vi "LanchSpeedAndAngleCalculator.vi"(2 "g":dbl=9.82, 3 "b":dbl=60.0, 4 "h":dbl, 5 "d":dbl) -> (0 "V":dbl, 1 "a":dbl)   [LabVIEW 2011]
uses:
  <vilib>/express/express arith-compare/Formula/XNode/ExpressFormulaBlockNode.xnode
panel:
  # "a - degrees\nb - degrees\nh - meters\nd - meters\ng - m/s^2\nV - m/s"
  # "b"
  # "V"
  # "h"
  # "a"
  # "d"
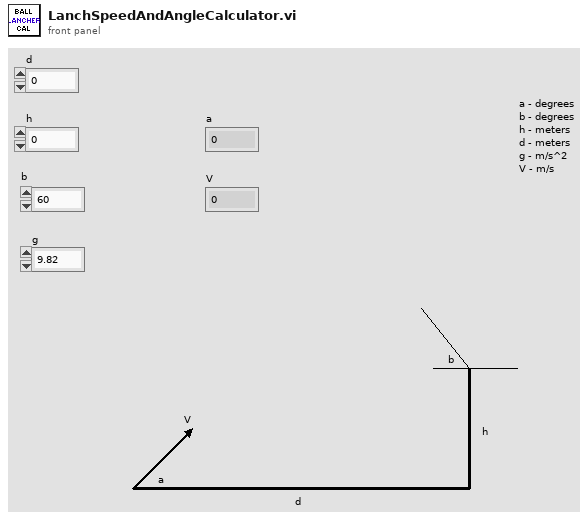
[diagram p1: front panel]
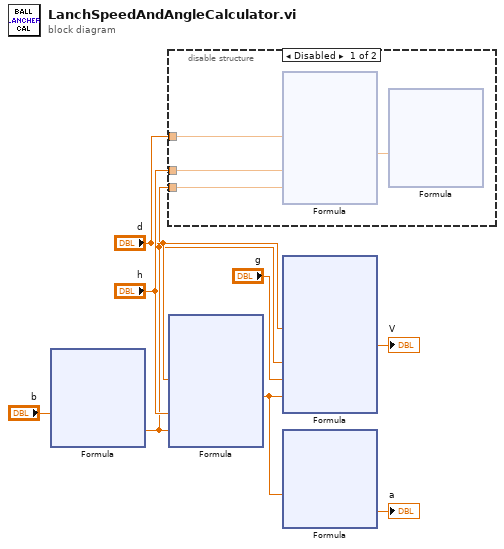
[diagram p0: block diagram]
diagram:
  n1 = xnode "Formula"("b"="b") -> ("Result"=w1:dbl)  [unwired: 1 in, 1 out]
  n2 = disable-structure shown="Disabled" {
    disable-tunnel: "d" -> [w12 _]
    disable-tunnel: "h" -> [w11 _]
    disable-tunnel: w1 -> [w10 _]
    frame Disabled {
      n3 = xnode "Formula"("d"=w12, "h"=w11, "b"=w10) -> ("Result"=w9:dbl)  [unwired: 1 in, 1 out]
      n4 = xnode "Formula"("r"=w9) -> ()  [unwired: 1 in, 2 out]
    }
    frame Enabled {
    }
  }
  n5 = xnode "Formula"("d"="d", "h"="h", "b"=w1) -> ("Result"=w3:dbl)  [unwired: 1 in, 1 out]
  n6 = xnode "Formula"("d"="d", "b"=w1, "g"="g", "a"=w3) -> ("Result"=→"V":dbl)  [unwired: 1 in, 1 out]
  n7 = xnode "Formula"("r"=w3) -> ("Result"=→"a":dbl)  [unwired: 1 in, 1 out]
